vi "testError.vi"(8 "error in (no error)":errorcluster) -> (0 "error out":errorcluster)   [LabVIEW 2019, in "AssertionTest.lvlib" / "AssertEquals.lvlib"]
uses:
  AssertEquals.lvlib
  AssertionTest.lvlib
  <vilib>/Utility/error.llb/Error Cluster From Error Code.vi
  <vilib>/ErrorRing/Error Ring.xnode
  Assertion/Assertion.lvlib
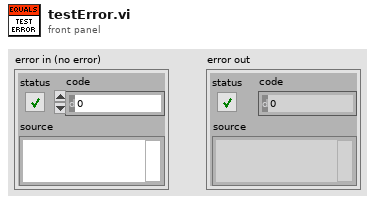
[diagram p1: front panel]
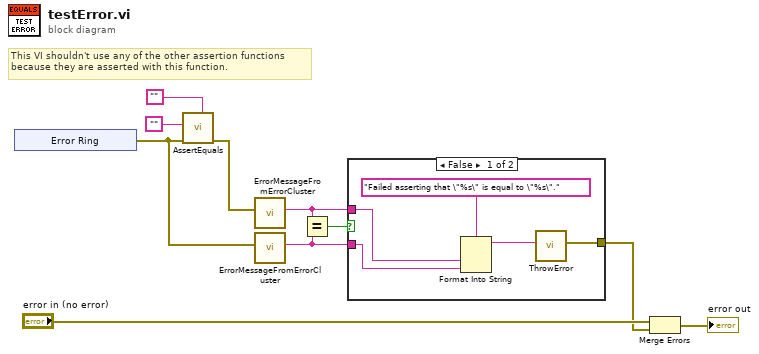
[diagram p0: block diagram]
diagram:
  # "This VI shouldn't use any of the other assertion functions\nbecause they are asserted with this function."
  n1 = xnode "Error Ring"() -> ("error out"=w10:errorcluster)
  n2 = call "AssertEquals.vi"("Expected"="", "error in (no error)"=w10, "Actual"="") -> ("error out"=w1:errorcluster)  [unwired: 8 in]
  n3 = call "ErrorMessageFromErrorCluster.vi"("Error"=w1) -> ("Error Message"=w8:string)  [unwired: 10 in]
  n4 = call "ErrorMessageFromErrorCluster.vi"("Error"=w10) -> ("Error Message"=w7:string)  [unwired: 10 in]
  n5 = Equal?(x=w8, y=w7) -> (x = y?=w9:bool)
  n6 = case shown="False" w9 {
    tunnel: w8 -> [w14 _]
    tunnel: w7 -> [w13 _]
    tunnel: [w11 _] -> w4
    frame False {
      n7 = Format Into String(format string="Failed asserting that \"%s\" is equal to \"%s\".", w14, w13) -> (resulting string=w12:string)  [unwired: 2 in, 1 out]
      n8 = call "ThrowError.vi"("Error Message"=w12) -> ("error out"=w11:errorcluster)  [unwired: 10 in]
    }
    frame True {
    }
  }
  n9 = Merge Errors("error in (no error)", w4) -> (→"error out":errorcluster)
